vi "GetGXMLCfgRTD.vi"(8 "error in (no error)":errorcluster, 11 "RTD in":refnum<class "RTD.lvclass">) -> (0 "error out":errorcluster, 2 "RTDChanCfg":T1, 3 "RTD out":refnum<class "RTD.lvclass">)   [LabVIEW 2012, in "Measurement Channels.lvlib" / "RTD.lvclass"]
uses:
  RTD.lvclass
  RTDProps_TD.ctl
  RTD.lvclass/RTD.ctl
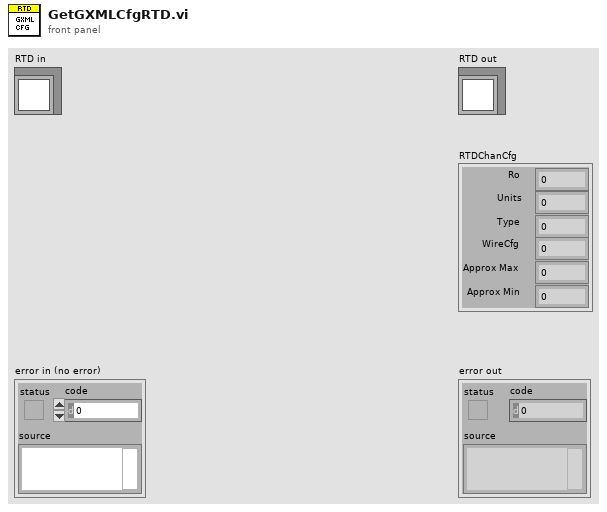
[diagram p1: front panel]
types:
  T1 = typedef "Measurement Channels.lvlib/RTD.lvclass/RTDProps_TD.ctl" = cluster{"Ro":u16, "Units":u16, "Type":u16, "WireCfg":u16, "Approx Max":dbl, "Approx Min":dbl}
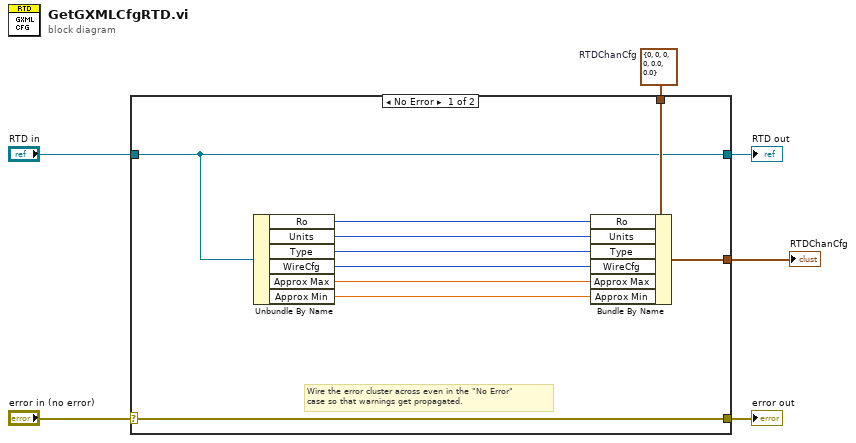
[diagram p0: block diagram]
diagram:
  w2 = T1 {"Ro"=0, "Units"=0, "Type"=0, "WireCfg"=0, "Approx Max"=0.0, "Approx Min"=0.0}  # RTDChanCfg
  n1 = case shown="No Error" "error in (no error)" {
    selector: "error in (no error)" -> [w16 w19]
    tunnel: [w16 w19] -> w5
    tunnel: [w13 w18] -> w3
    tunnel: "RTD in" -> [w13 w18]
    tunnel: w2 -> [w15 w17]
    tunnel: [w14 w17] -> w1
    frame No Error {
      # "Wire the error cluster across even in the \"No Error\"\ncase so that warnings get propagated."
      n2 = Unbundle By Name(w13) -> ("Ro"=w12:u16, "Units"=w11:u16, "Type"=w10:u16, "WireCfg"=w9:u16, "Approx Max"=w8:dbl, "Approx Min"=w7:dbl)
      n3 = Bundle By Name(cluster=w15, "Ro"=w12, "Units"=w11, "Type"=w10, "WireCfg"=w9, "Approx Max"=w8, "Approx Min"=w7) -> (w14:T1)
    }
    frame Error {
    }
  }
  "error out" <- w5
  "RTD out" <- w3
  "RTDChanCfg" <- w1
